vi "GetParent__slk_tc.vi"(0 "tree control in":refnum<class "TreeControl.lvclass">, 5 "child tag (\"\")":string, 11 "error in (no error)":errorcluster) -> (4 "tree control out":refnum<class "TreeControl.lvclass">, 6 "parent tag":string, 10 "parents tags":string[](array[string]), 15 "error out":errorcluster)   [LabVIEW 2020, in "TreeControl.lvclass"]
doc: "Retrieves the parent of the input child or the currently selected item . Also returns a 1-D array of all members in its family starting at its parent and leading back to its most mature member."
uses:
  Library/TreeControl.lvclass
  Library/TreeControl.lvclass/TreeControl.ctl
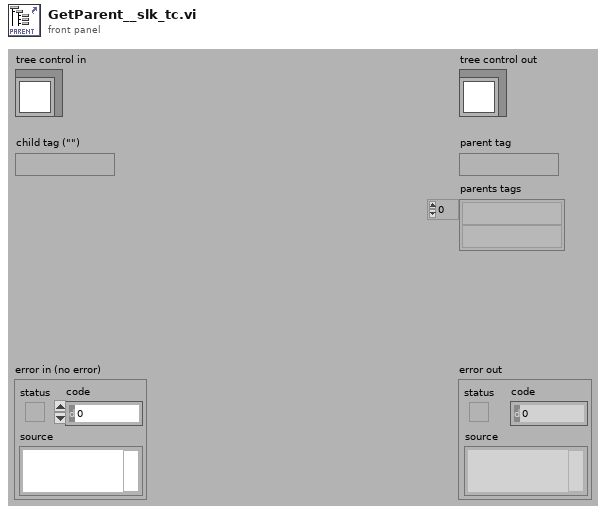
[diagram p1: front panel]
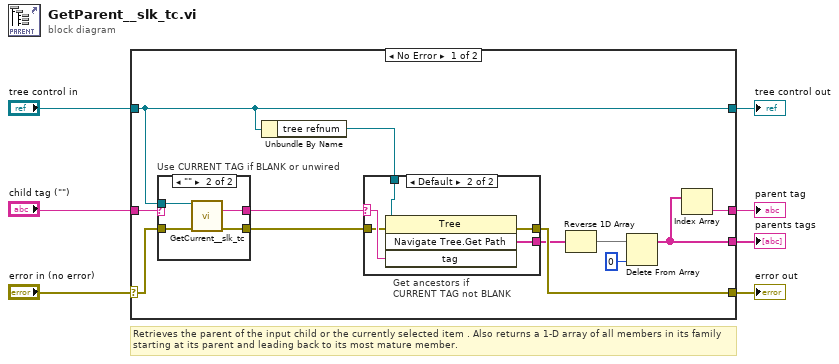
[diagram p0: block diagram]
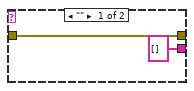
[diagram p2: hidden frame]
diagram:
  # "Retrieves the parent of the input child or the currently selected item . Also returns a 1-D array of all members in its family starting at its parent and leading back to its most mature member."
  n1 = case shown="No Error" "error in (no error)" {
    selector: "error in (no error)" -> [w14 w34]
    tunnel: [w13 w34] -> w6
    tunnel: [w18 w33] -> w4
    tunnel: "tree control in" -> [w18 w33]
    tunnel: "child tag (\"\")" -> [w19 _]
    tunnel: [w8 _] -> w2
    tunnel: [w9 _] -> w1
    frame No Error {
      n2 = case "Use CURRENT TAG if BLANK or unwired" shown="\"\"" w19 {
        selector: w19 -> [w28 _]
        tunnel: [w28 w32] -> w17
        tunnel: w18 -> [_ w31]
        tunnel: w14 -> [w27 w30]
        tunnel: [w27 w29] -> w15
        frame Default {
        }
        frame "" {
          n3 = call "GetCurrent__slk_tc.vi"("tree control in"=w31, "error in (no error)"=w30) -> ("current tag"=w32:string, "error out"=w29:errorcluster)  [unwired: 1 in, 11 out]
        }
      }
      n4 = Unbundle By Name(w18) -> ("tree refnum"=w16:refnum<vi>)
      n5 = case "Get ancestors if CURRENT TAG not BLANK" shown="Default" w17 {
        selector: w17 -> [_ w26]
        tunnel: w16 -> [_ w25]
        tunnel: [string[] [] ("Navigate Tree:Get Path") w24] -> w12
        tunnel: w15 -> [w21 w23]
        tunnel: [w21 w22] -> w13
        frame "" {
        }
        frame Default {
          n6 = invoke class="Tree" method="Navigate Tree.Get Path"(reference=w25, error in=w23, "tag"=w26) -> (error out=w22:errorcluster, "Navigate Tree:Get Path"=w24:string[])  [unwired: 1 in, 2 out]
        }
      }
      n7 = Reverse 1D Array(array=w12) -> (reversed array=w10:string[])
      n8 = Delete From Array(array=w10, index=0) -> (array with subset deleted=w8:string[])  [unwired: 1 in, 1 out]
      n9 = Index Array(array=w8) -> (element=w9:string)  [unwired: 1 in]
    }
    frame Error {
    }
  }
  "error out" <- w6
  "tree control out" <- w4
  "parent tag" <- w1
  "parents tags" <- w2
